vi "Get Tags.vi"(8 "error in (no error)":errorcluster, 11 "eLab in":refnum<class "PL eLabFTW Client.lvclass">) -> (0 "error out":errorcluster, 2 "tags":cluster{"id":u32, "name":string}[](array[cluster]), 3 "eLab out":refnum<class "PL eLabFTW Client.lvclass">)   [LabVIEW 2015, in "PL eLabFTW Client.lvclass"]
doc: "Gets tags."
uses:
  PL eLabFTW Client.lvclass
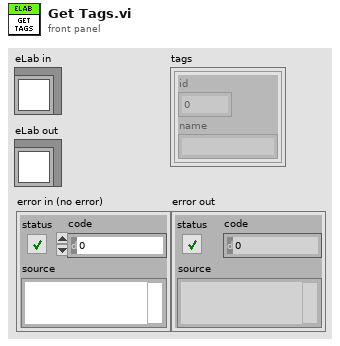
[diagram p1: front panel]
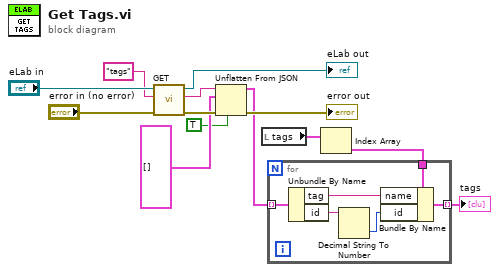
[diagram p0: block diagram]
diagram:
  n1 = call "GET.vi"("error in (no error)"="error in (no error)", "relative URL"="tags", "eLab in"="eLab in") -> ("error out"=w8:errorcluster, "response body"=w9:string, "eLab out"=→"eLab out":refnum<class "PL eLabFTW Client.lvclass">)  [unwired: 6 in]
  n2 = Unflatten From JSON(JSON string=w9, type and defaults=cluster{"tag":string, "id":string}[] [], default null elements? (F)=TRUE, error in (no error)=w8) -> (value=w5:cluster{"tag":string, "id":string}[], error out=→"error out":errorcluster)  [unwired: 3 in]
  n3 = local read "tags"() -> (w4:cluster{"id":u32, "name":string}[])
  n4 = Index Array(array=w4) -> (element=w3:cluster{"id":u32, "name":string})  [unwired: 1 in]
  n5 = for {
    tunnel: w5 -> [w19] mode=indexing
    tunnel: w3 -> [w17]
    tunnel: [w14] -> w2 mode=indexing
    n6 = Unbundle By Name(w19) -> ("tag"=w16:string, "id"=w18:string)
    n7 = Decimal String To Number(string=w18) -> (number=w15:i32)  [unwired: 2 in, 1 out]
    n8 = Bundle By Name(cluster=w17, "name"=w16, "id"=w15) -> (w14:cluster{"id":u32, "name":string})
  }
  "tags" <- w2
